vi "Increment_Step_Duration.vi"(8 "error in (no error)":errorcluster, 11 "Data Cluster in":T1) -> (0 "error out":errorcluster, 3 "Data Cluster out":T1)   [LabVIEW 2026]
uses:
  controls/UI Data.ctl
  controls/Display_Panel.ctl
  controls/Controls.ctl
  controls/Program_Settings.ctl
  controls/System_State.ctl
  controls/Mode.ctl
panel:
  # "Manual Setting"
  # "Manual Setting"
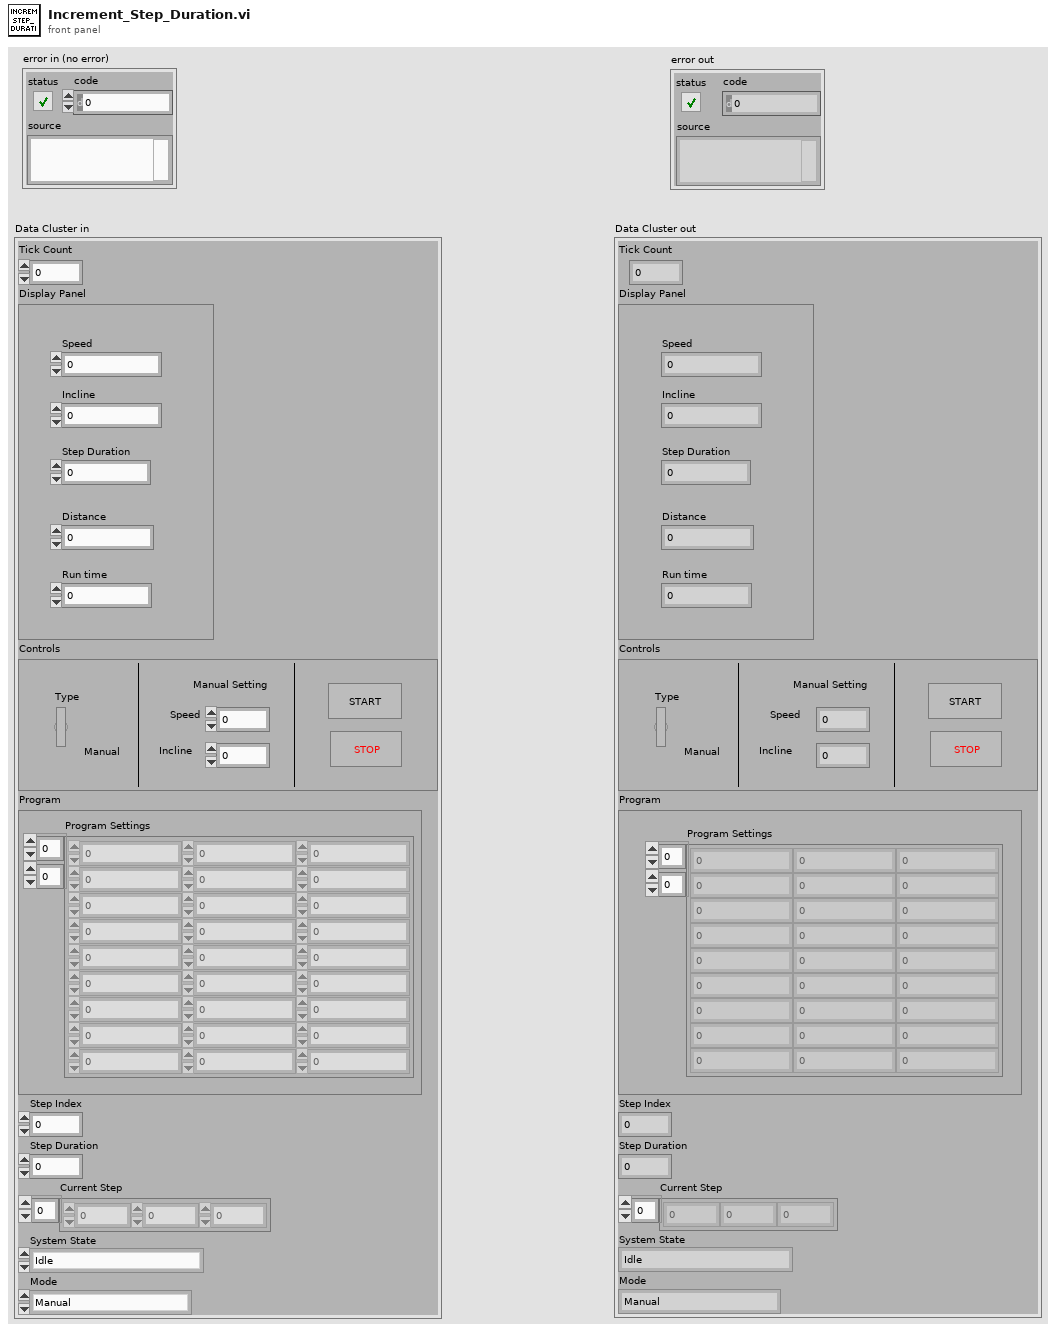
[diagram p1: front panel]
types:
  T1 = typedef "UI Data.ctl" = cluster{"Tick Count":dbl, "Display Panel":T2, "Controls":T3, "Program":T4, "Step Index":u32, "Step Duration":dbl, "Current Step":dbl[], "System State":T5, "Mode":T6}
  T2 = typedef "Display_Panel.ctl" = cluster{"Speed":dbl, "Incline":dbl, "Step Duration":dbl, "Distance":dbl, "Run time":dbl}
  T3 = typedef "Controls.ctl" = cluster{"Type":bool, "Speed":dbl, "Incline":dbl, "Start":bool, "stop":bool}
  T4 = typedef "Program_Settings.ctl" = cluster{"Program Settings":dbl[][]}
  T5 = typedef "System_State.ctl" = enum16{"Idle", "Running", "Ramp_Down"}
  T6 = typedef "Mode.ctl" = enum16{"Manual", "Program"}
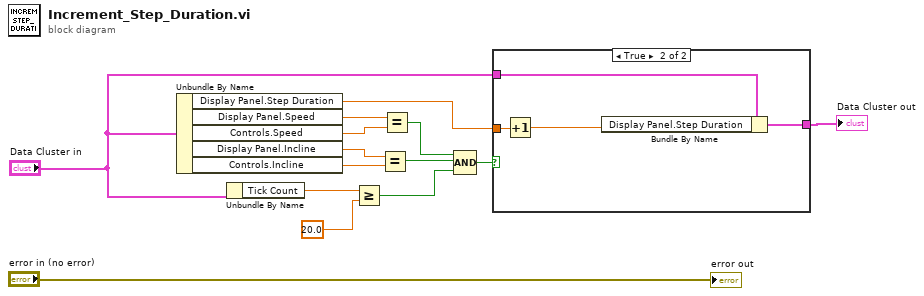
[diagram p0: block diagram]
diagram:
  n1 = Unbundle By Name("Data Cluster in") -> ("Display Panel.Step Duration"=w3:dbl, "Display Panel.Speed"=w13:dbl, "Controls.Speed"=w12:dbl, "Display Panel.Incline"=w11:dbl, "Controls.Incline"=w10:dbl)
  n2 = Unbundle By Name("Data Cluster in") -> ("Tick Count"=w8:dbl)
  n3 = Greater Or Equal?(x=w8, y=20.0) -> (x >= y?=w7:bool)
  n4 = Equal?(x=w11, y=w10) -> (x = y?=w5:bool)
  n5 = Equal?(x=w13, y=w12) -> (x = y?=w6:bool)
  n6 = Compound Arithmetic op=AND(w6, w5, w7) -> (w4:bool)
  n7 = case shown="True" w4 {
    tunnel: w3 -> [_ w19]
    tunnel: "Data Cluster in" -> [w15 w18]
    tunnel: [w15 w16] -> w1
    frame False {
    }
    frame True {
      n8 = Increment(x=w19) -> (x+1=w17:dbl)
      n9 = Bundle By Name(cluster=w18, "Display Panel.Step Duration"=w17) -> (w16:T1)
    }
  }
  "Data Cluster out" <- w1
  "error out" <- "error in (no error)"
